vi "DOCK_create_queues.vi"(8 "error_in":errorcluster, 11 "all_config_info_in":T1={"main_ini_file"={"SQL Driver"="", "SQL Server"="", "SQL Database"="", "SQL UID"="", "Reference table"="", "Reference history"="", "Archivisation CFG table"="", "Archivisation CFG history"="", "User table"="", "User history"="", "default language"="", "SCANNER COM port"=0, "SCANNER Baud rate"=0, "SCANNER Data bits"=0, "SCANNER Pairity"=enum."None", "SCANNER Stop bits"=0, "SCANNER Flow control"=0, "SCANNER Termination char"=10, "PRINTER PC port"=0, "PRINTER IP"="", "PRINTER port"=0, "PRINTER Keep alive timer [ms]"=0, "logout timeout [ms]"=0}, "SQL Password"="", "PRINTER Label"="", "PRINTER Template"="", "Last Label"="", "queue_refnums"={"MAIN_queue"=refnum, "SCANNER_queue"=refnum, "SCANNER_login"=refnum, "PRINTER_queue"=refnum}} {"main_ini_file"."SCANNER Flow control" items=["None"=0, "XON/XOFF"=1, "RTS/CTS"=2, "DTR/DSR"=4]; "main_ini_file"."SCANNER Stop bits" items=["1.0"=10, "1.5"=15, "2.0"=20]}) -> (0 "error_out":errorcluster, 3 "all_config_info_out":T1={"main_ini_file"={"SQL Driver"="", "SQL Server"="", "SQL Database"="", "SQL UID"="", "Reference table"="", "Reference history"="", "Archivisation CFG table"="", "Archivisation CFG history"="", "User table"="", "User history"="", "default language"="", "SCANNER COM port"=0, "SCANNER Baud rate"=0, "SCANNER Data bits"=0, "SCANNER Pairity"=enum."None", "SCANNER Stop bits"=0, "SCANNER Flow control"=0, "SCANNER Termination char"=10, "PRINTER PC port"=0, "PRINTER IP"="", "PRINTER port"=0, "PRINTER Keep alive timer [ms]"=0, "logout timeout [ms]"=0}, "SQL Password"="", "PRINTER Label"="", "PRINTER Template"="", "Last Label"="", "queue_refnums"={"MAIN_queue"=refnum, "SCANNER_queue"=refnum, "SCANNER_login"=refnum, "PRINTER_queue"=refnum}} {"main_ini_file"."SCANNER Flow control" items=["None"=0, "XON/XOFF"=1, "RTS/CTS"=2, "DTR/DSR"=4]; "main_ini_file"."SCANNER Stop bits" items=["1.0"=10, "1.5"=15, "2.0"=20]})   [LabVIEW 2019]
uses:
  ini/typedef/DOCK_all_config_info.ctl
  ini/typedef/DOCK_main_ini_file.ctl
  typedef/DOCK_queue_refnums.ctl
  typedef/DOCK_MAIN_queue_element.ctl
  MAIN/DOCK_MAIN_sequence_state.ctl
  typedef/DOCK_SCANNER_queue_element.ctl
  SCANNER/DOCK_SCANNER_sequence_state.ctl
  typedef/DOCK_PRINTER_queue_element.ctl
  PRINTER/DOCK_PRINTER_sequence_state.ctl
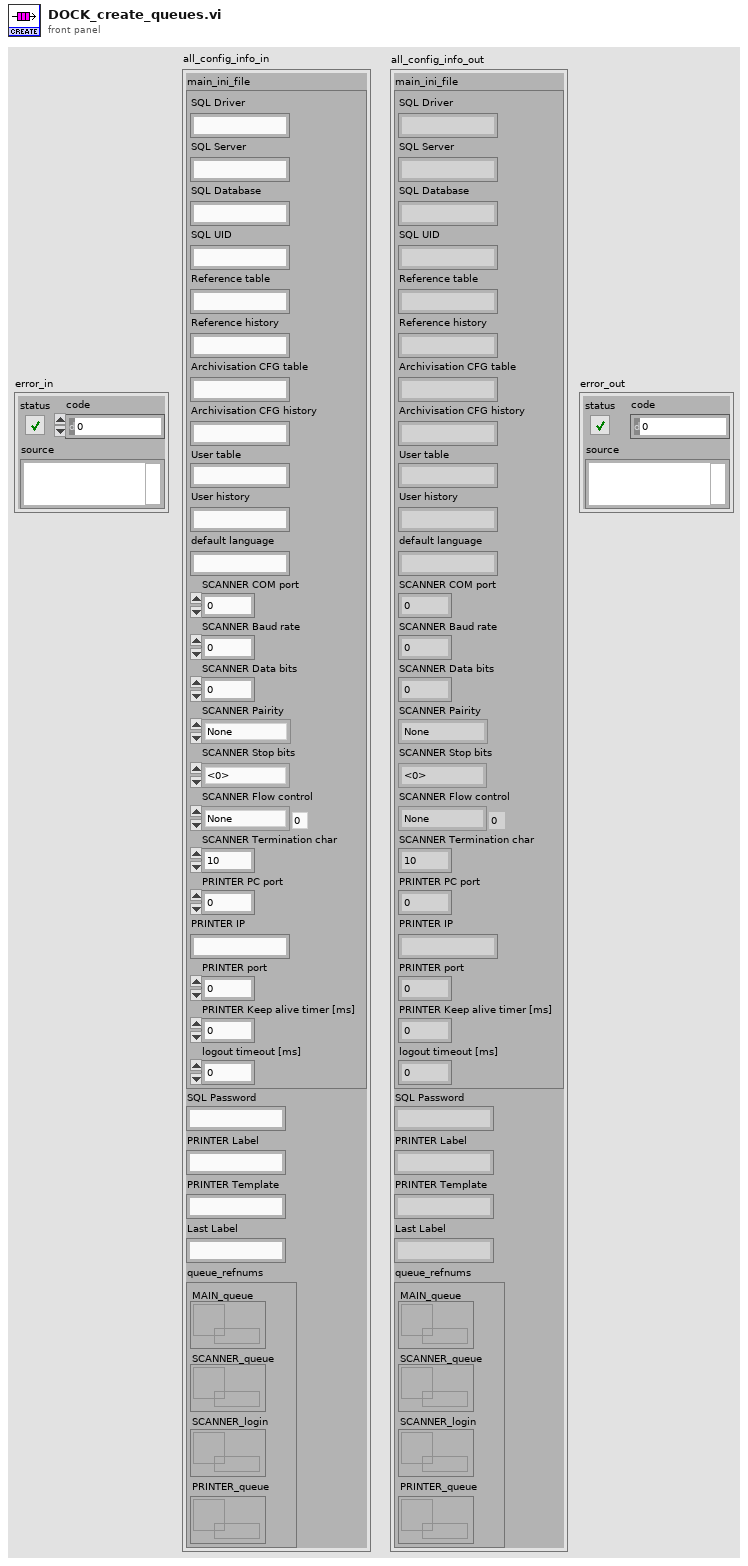
[diagram p1: front panel]
types:
  T1 = typedef "DOCK_all_config_info.ctl" = cluster{"main_ini_file":T2, "SQL Password":string, "PRINTER Label":string, "PRINTER Template":string, "Last Label":string, "queue_refnums":T3}
  T2 = typedef "DOCK_main_ini_file.ctl" = cluster{"SQL Driver":string, "SQL Server":string, "SQL Database":string, "SQL UID":string, "Reference table":string, "Reference history":string, "Archivisation CFG table":string, "Archivisation CFG history":string, "User table":string, "User history":string, "default language":string, "SCANNER COM port":u16, "SCANNER Baud rate":u32, "SCANNER Data bits":u16, "SCANNER Pairity":enum16{"None", "Odd", "Even", "Mark", "Space"}, "SCANNER Stop bits":u16, "SCANNER Flow control":u16, "SCANNER Termination char":u8, "PRINTER PC port":u16, "PRINTER IP":string, "PRINTER port":u16, "PRINTER Keep alive timer [ms]":i32, "logout timeout [ms]":i32}
  T3 = typedef "DOCK_queue_refnums.ctl" = cluster{"MAIN_queue":refnum<queue>, "SCANNER_queue":refnum<queue>, "SCANNER_login":refnum<queue>, "PRINTER_queue":refnum<queue>}
  T4 = typedef "DOCK_PRINTER_queue_element.ctl" = cluster{"state":T5, "variable":variant}
  T5 = typedef "DOCK_PRINTER_sequence_state.ctl" = enum16{"initialize", "get_next_state", "send", "keep_alive", "error", "stop"}
  T6 = typedef "DOCK_SCANNER_queue_element.ctl" = cluster{"state":T7, "variable":variant}
  T7 = typedef "DOCK_SCANNER_sequence_state.ctl" = enum16{"initialize", "get_next_state", "read", "error", "stop"}
  T8 = typedef "DOCK_MAIN_queue_element.ctl" = cluster{"state":T9, "variable":variant}
  T9 = typedef "DOCK_MAIN_sequence_state.ctl" = enum16{"initialize", "get_next_state", "USER_login", "USER_logout", "read_reference_list", "read_batch_size_list", "change_reference", "start_batch", "reload_batch", "finish_batch?", "finish_batch", "preread_gear_data_check", "read_gear_data", "refresh_gear_data", "save_gear_to_batch", "clear_gear_data", "print_label", "report_get", "error", "stop"}
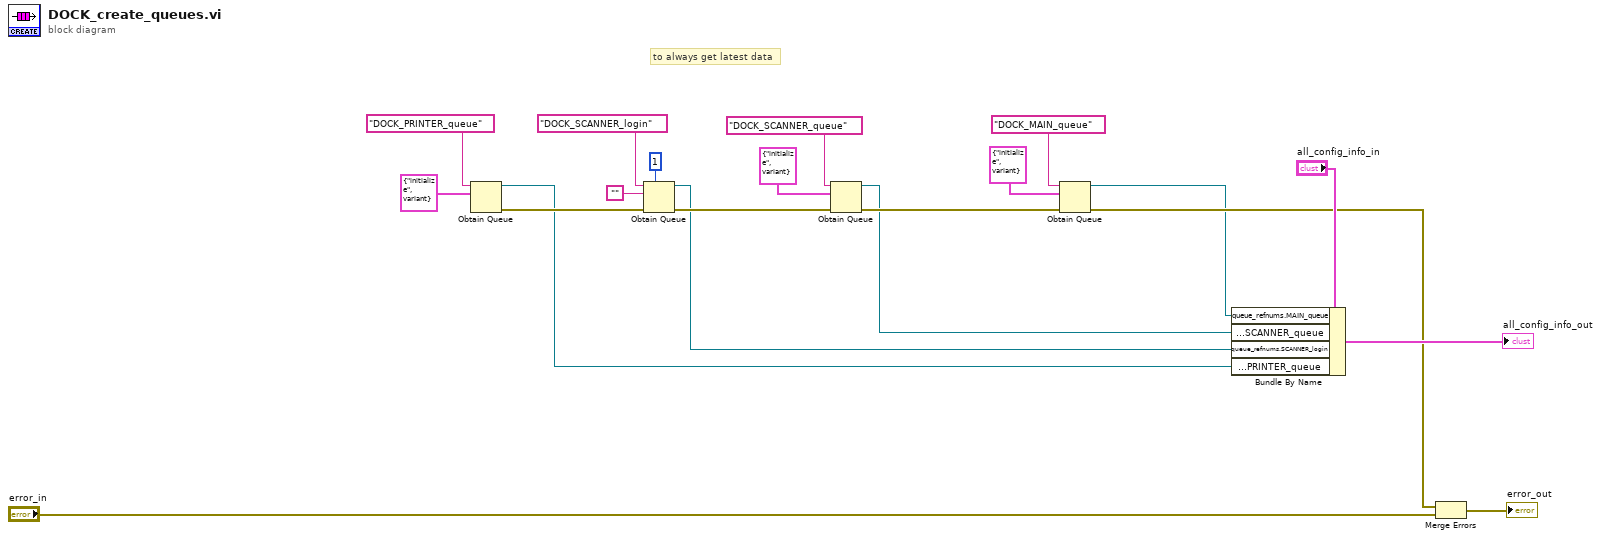
[diagram p0: block diagram]
diagram:
  # "to always get latest data"
  n1 = Obtain Queue(name (unnamed)="DOCK_PRINTER_queue", element data type=T4 {"state"=enum."initialize", "variable"=variant} ("DOCK_PRINTER_queue_element")) -> (queue out=w1:refnum<queue>, error out=w3:errorcluster)  [unwired: 3 in, 1 out]
  n2 = Obtain Queue(max queue size (-1, unlimited)=1, name (unnamed)="DOCK_SCANNER_login", element data type="", error in (no error)=w3) -> (queue out=w9:refnum<queue>, error out=w12:errorcluster)  [unwired: 1 in, 1 out]
  n3 = Obtain Queue(name (unnamed)="DOCK_SCANNER_queue", element data type=T6 {"state"=enum."initialize", "variable"=variant} ("DOCK_SCANNER_queue_element"), error in (no error)=w12) -> (queue out=w7:refnum<queue>, error out=w15:errorcluster)  [unwired: 2 in, 1 out]
  n4 = Obtain Queue(name (unnamed)="DOCK_MAIN_queue", element data type=T8 {"state"=enum."initialize", "variable"=variant} ("DOCK_MAIN_queue_element"), error in (no error)=w15) -> (queue out=w5:refnum<queue>, error out=w16:errorcluster)  [unwired: 2 in, 1 out]
  n5 = Bundle By Name(cluster="all_config_info_in", "queue_refnums.MAIN_queue"=w5, "queue_refnums.SCANNER_queue"=w7, "queue_refnums.SCANNER_login"=w9, "queue_refnums.PRINTER_queue"=w1) -> (→"all_config_info_out":T1)
  n6 = Merge Errors(w16, "error_in") -> (→"error_out":errorcluster)
